vi "Mark as Source Only.vi"() -> ()   [LabVIEW 2011]
uses:
  <vilib>/regexp/Match Regular Expression.xnode
panel:
  out "Array":path[](array[path])
  out "Progess":i32(slide) scale=0.0..20.0
  in  "Mark VIs":bool
  in  "IgnoreSVN":bool=TRUE
  in  "Root Folder":path
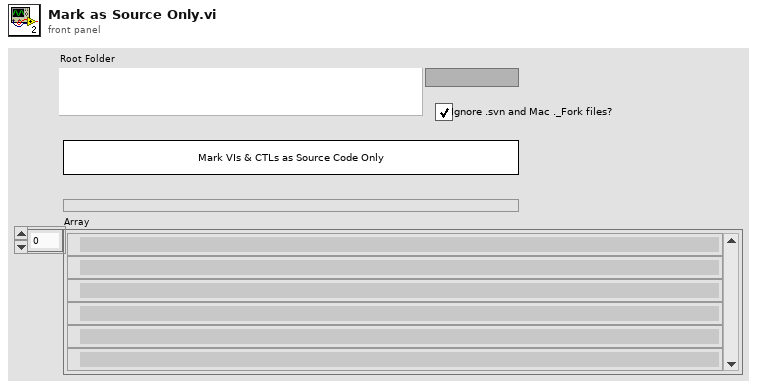
[diagram p1: front panel]
types:
  T1 = enum32{"invalid VI type", "Standard VI", "Control VI", "Global VI", "Polymorphic VI", "Configuration VI", "SubSystem", "Facade VI", "Method VI", "Statechart Diagram VI"}[]
  T2 = enum32{"invalid VI type", "Standard VI", "Control VI", "Global VI", "Polymorphic VI", "Configuration VI", "SubSystem", "Facade VI", "Method VI", "Statechart Diagram VI"}
  T3 = enum16{"Left Button", "Center Button", "Right Button", "Window Close"}
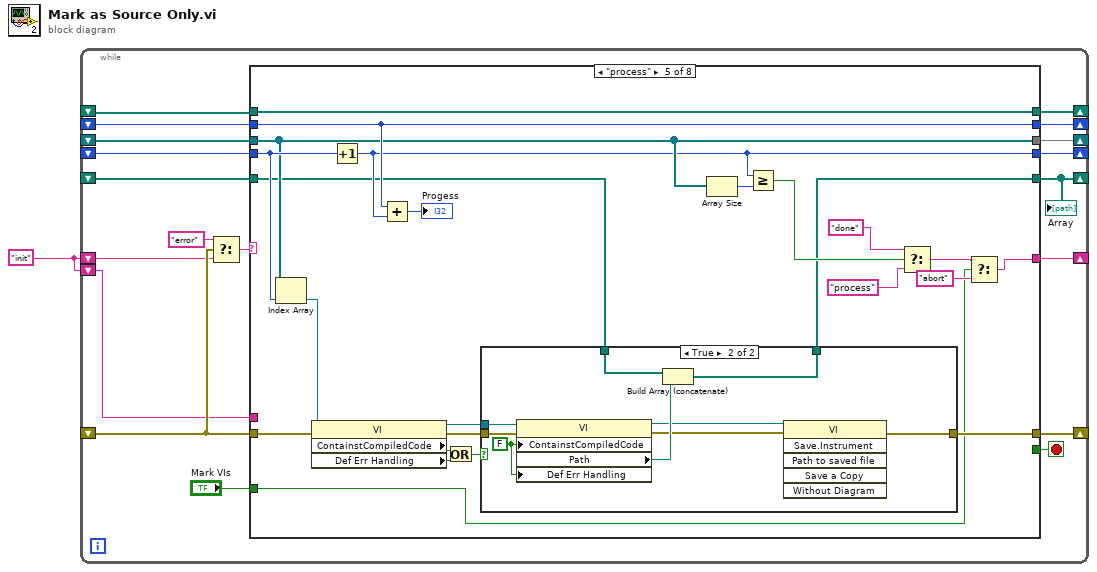
[diagram p0: block diagram]
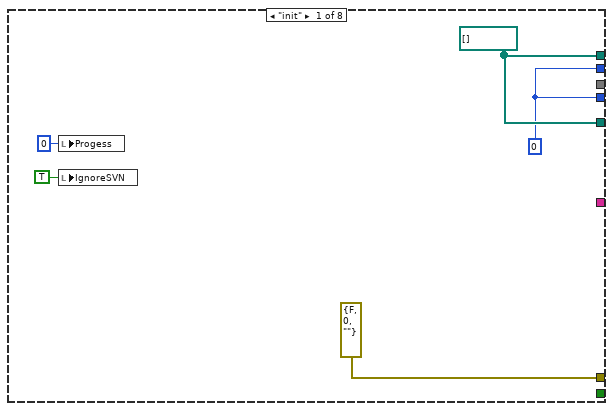
[diagram p2: hidden frame]
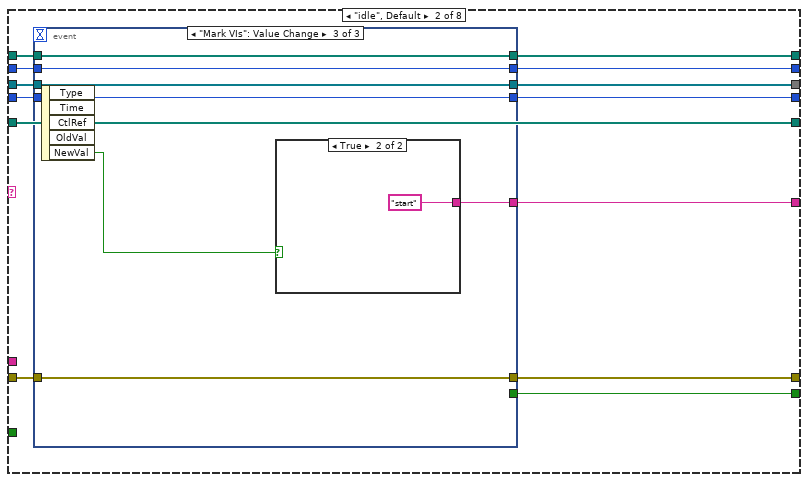
[diagram p3: hidden frame]
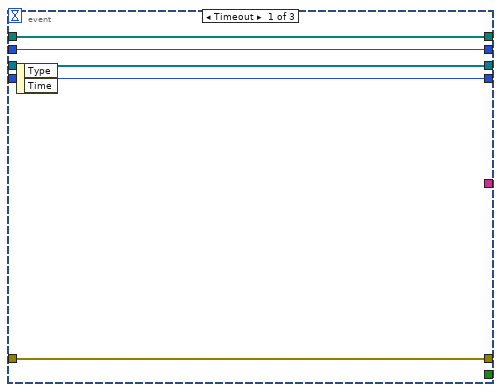
[diagram p4: hidden frame]
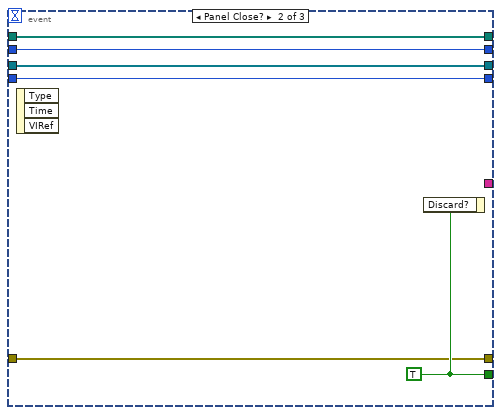
[diagram p5: hidden frame]
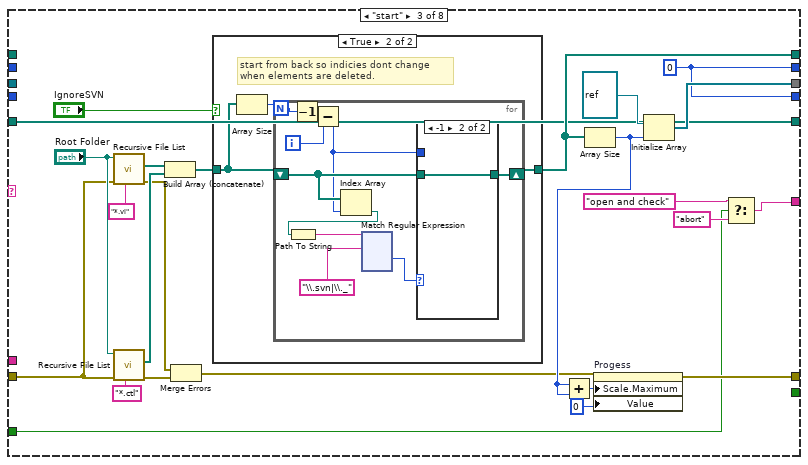
[diagram p7: hidden frame]
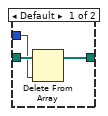
[diagram p9: hidden frame]
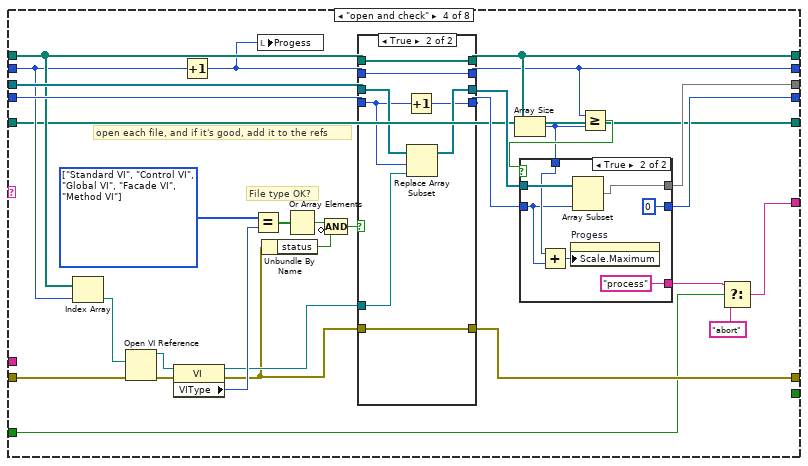
[diagram p10: hidden frame]
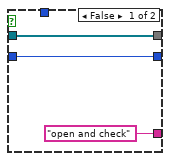
[diagram p11: hidden frame]
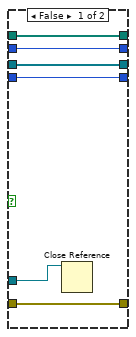
[diagram p12: hidden frame]
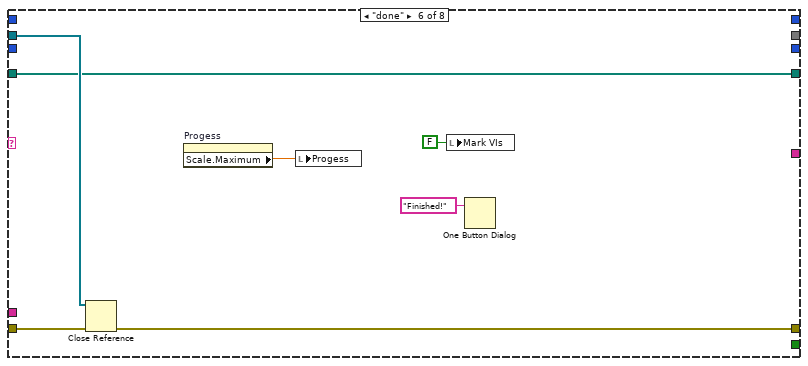
[diagram p14: hidden frame]
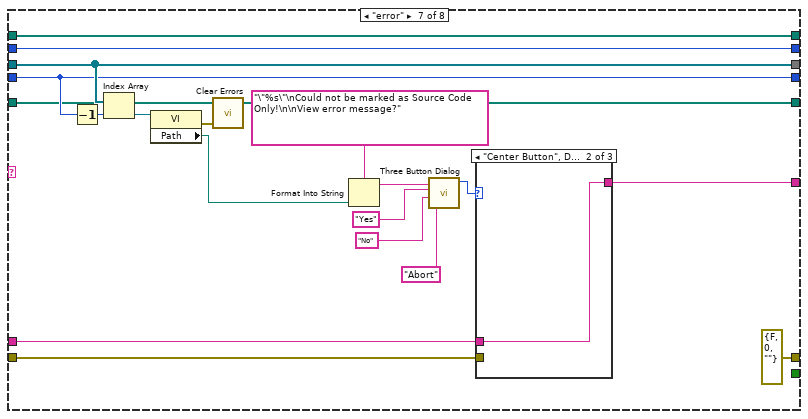
[diagram p15: hidden frame]
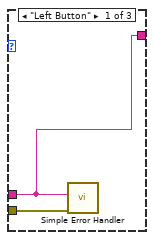
[diagram p16: hidden frame]
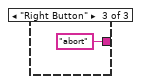
[diagram p17: hidden frame]
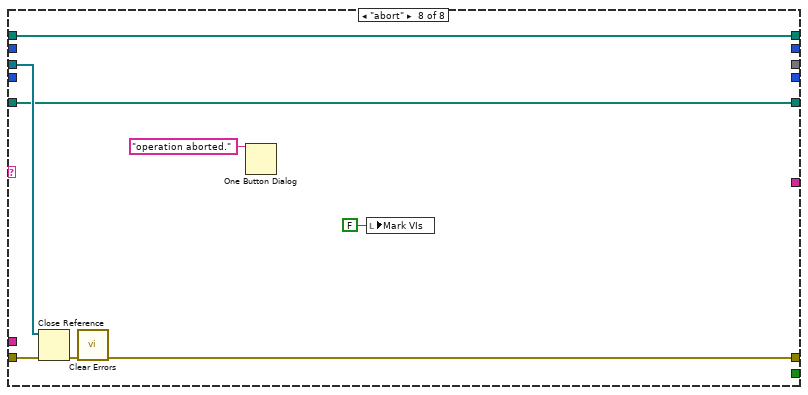
[diagram p18: hidden frame]
diagram:
  w1 = "init"
  n1 = while {
    shift-right: [w15] -> _
    shift-left: w1 -> [w4]
    shift-right: [w16] -> _
    shift-left: _ -> [w17]
    shift-right: [w14] -> _
    shift-left: _ -> [w13]
    shift-right: [w11] -> _
    shift-left: _ -> [w12]
    shift-right: [w10] -> _
    shift-left: _ -> [w9]
    shift-right: [w7] -> _
    shift-left: _ -> [w8]
    shift-left: w1 -> [w5]
    shift-right: [w2] -> _
    shift-left: _ -> [w3]
    stop <- w20 stop-if-true
    n2 = Select(t="error", s=w17, f=w4) -> (s? t:f=w18:string)
    n3 = case shown="\"process\"" w18 {
      tunnel: [_ w38 _ _ _ _ _ _] -> w20
      tunnel: w17 -> [_ w37 w67 w241 w273 w307 w317 w335]
      tunnel: [errorcluster {"status"=FALSE, "code"=0, "source"=""} ("error in") w36 w76 w227 w285 w305 errorcluster {"status"=FALSE, "code"=0, "source"=""} ("error out") w333] -> w16
      tunnel: [_ w35 w60 w213 w277 _ w312 _] -> w15
      tunnel: [w23 w32 w63 w224 w286 _ w326 w332] -> w14
      tunnel: w13 -> [_ w34 _ w228 w286 _ w326 w332]
      tunnel: w12 -> [_ w33 _ w225 w287 _ w325 _]
      tunnel: [w22 w31 w70 w220 w287 _ w325 _] -> w11
      tunnel: [_ w30 w73 w218 w284 _ w323 _] -> w10
      tunnel: w9 -> [_ w29 _ w234 w284 w306 w323 w336]
      tunnel: w8 -> [_ w28 _ w232 w289 _ w311 _]
      tunnel: [w22 w27 w70 w221 w282 _ w311 _] -> w7
      tunnel: "Mark VIs" -> [_ _ w59 w215 w275 _ _ _]
      tunnel: w5 -> [_ _ _ _ _ _ w309 _]
      tunnel: w3 -> [_ w26 w58 w211 w270 w301 w308 w331]
      tunnel: [w23 w26 w58 w211 w269 w301 w308 w331] -> w2
      frame "init" {
        w22 = 0
        w23 = path[] []
        n4 = local write "Progess"(0 ("Progess")) -> ()
        n5 = local write "IgnoreSVN"(TRUE ("IgnoreSVN")) -> ()
      }
      frame "idle", Default {
        n6 = event shown="[2] \"Mark VIs\": Value Change" {
          selector: _ -> [_ _ _]
          dyn-events: _ -> [_ _ _]
          timeout: _ -> [_ _ _]
          tunnel: [_ w49 _] -> w38
          tunnel: w37 -> [w43 w48 w56]
          tunnel: [w43 w48 w56] -> w36
          tunnel: [_ _ w55] -> w35
          tunnel: w34 -> [w41 w47 w53]
          tunnel: w33 -> [w42 w46 w54]
          tunnel: [w41 w47 w53] -> w32
          tunnel: [w42 w46 w54] -> w31
          tunnel: [w39 w45 w51] -> w30
          tunnel: w29 -> [w39 w45 w51]
          tunnel: w28 -> [w40 w44 w52]
          tunnel: [w40 w44 w52] -> w27
          event Timeout {
            n7 = event-data() -> ()  [unwired: 1 in, 2 out]
          }
          event Panel Close? {
            w49 = TRUE
            n8 = event-data() -> ()  [unwired: 1 in, 3 out]
            n9 = event-data("Discard?"=w49) -> ()  [unwired: 1 in, 1 out]
          }
          event "Mark VIs": Value Change {
            n10 = event-data() -> ("NewVal"=w50:bool)  [unwired: 1 in, 4 out]
            n11 = case shown="True" w50 {
              tunnel: [_ "start"] -> w55
              frame False {
              }
              frame True {
              }
            }
          }
        }
      }
      frame "start" {
        w70 = 0
        n12 = call <vilib>:"Recursive File List.vi"("pattern"="*.vi", "error in (no error)"=w67, "Folder Path"="Root Folder") -> ("error out"=w68:errorcluster, "All Files in Dir"=w78:path[])  [unwired: 4 in, 3 out]
        n13 = call <vilib>:"Recursive File List.vi"("pattern"="*.ctl", "error in (no error)"=w67, "Folder Path"="Root Folder") -> ("error out"=w66:errorcluster, "All Files in Dir"=w77:path[])  [unwired: 4 in, 3 out]
        n14 = Build Array (concatenate)(w78, w77) -> (w69:path[])
        n15 = Merge Errors(w68, w66) -> (w65:errorcluster)
        n16 = case shown="True" "IgnoreSVN" {
          tunnel: w69 -> [w82 w83]
          tunnel: [w82 w85] -> w63
          frame False {
          }
          frame True {
            # "start from back so indicies dont change\nwhen elements are deleted."
            n17 = Array Size(array=w83) -> (size(s)=w84:i32)
            n18 = for {
              N: w84 -> [w95]
              shift-right: [w90] -> w85
              shift-left: w83 -> [w92]
              i -> [w94]
              n19 = Decrement(x=w95) -> (x-1=w89:i32)
              n20 = Subtract(x=w89, y=w94) -> (x-y=w91:i32)
              n21 = Index Array(array=w92, index=w91) -> (element=w93:path)
              n22 = Path To String(path=w93) -> (string=w88:string)
              n23 = xnode "Match Regular Expression"("input string"=w88, "regular expression"="\\.svn|\\._") -> ("offset past match"=w87:i32)  [unwired: 4 in, 4 out]
              n24 = case shown="-1" w87 {
                tunnel: w92 -> [w209 w210]
                tunnel: w91 -> [w207 _]
                tunnel: [w208 w210] -> w90
                frame Default {
                  n25 = Delete From Array(array=w209, index=w207) -> (array with subset deleted=w208:path[])  [unwired: 1 in, 1 out]
                }
                frame -1 {
                }
              }
            }
          }
        }
        n26 = Array Size(array=w63) -> (size(s)=w71:i32)
        n27 = Add(x=w71, y=w71) -> (x+y=w72:i32)
        n28 = property on="Progess" class="Slide (strict)"(error in=w65, "Scale.Maximum"=w72, "Value"=0 ("Progess")) -> (error out=w76:errorcluster)  [unwired: 1 in, 1 out]
        n29 = Initialize Array(refnum<vi> refnum ("This VI"), w71) -> (w73:refnum<vi>[])
        n30 = Select(t="open and check", s=w59, f="abort") -> (s? t:f=w60:string)
      }
      frame "open and check" {
        w236 = T1 [enum."Standard VI", enum."Control VI", enum."Global VI", enum."Facade VI", enum."Method VI"] items=["invalid VI type", "Standard VI", "Control VI", "Global VI", "Polymorphic VI", "Configuration VI", "SubSystem", "Facade VI", "Method VI", "Statechart Diagram VI"]
        # "open each file, and if it's good, add it to the refs"
        # "File type OK?"
        n31 = Index Array(array=w228, index=w225) -> (element=w240:path)
        n32 = Open VI Reference(vi path=w240, error in (no error)=w241) -> (vi reference=w238:refnum<vi>, error out=w239:errorcluster)  [unwired: 4 in]
        n33 = property class="VI"(reference=w238, error in=w239) -> (reference out=w233:refnum<vi>, error out=w226:errorcluster, "VIType"=w237:T2)
        n34 = Increment(x=w225) -> (x+1=w219:i32)
        n35 = Equal?(x=w236, y=w237) -> (x = y?=w235:bool[])
        n36 = local write "Progess"(w219) -> ()
        n37 = Unbundle By Name(w226) -> ("status"=w230:bool)
        n38 = Or Array Elements(Boolean array=w235) -> (logical OR=w231:bool)
        n39 = Compound Arithmetic op=AND(w231, invert w230) -> (w229:bool)
        n40 = case shown="True" w229 {
          tunnel: w234 -> [w255 w265]
          tunnel: w233 -> [w253 w264]
          tunnel: [w255 w263] -> w222
          tunnel: w232 -> [w254 w262]
          tunnel: [w254 w261] -> w217
          tunnel: w228 -> [w257 w260]
          tunnel: [w257 w260] -> w224
          tunnel: [w256 w259] -> w220
          tunnel: w219 -> [w256 w259]
          tunnel: [w252 w258] -> w227
          tunnel: w226 -> [w252 w258]
          frame False {
            n41 = Close Reference(reference=w253) -> ()  [unwired: 1 in, 1 out]
          }
          frame True {
            n42 = Increment(x=w262) -> (x+1=w261:i32)
            n43 = Replace Array Subset(array=w265, new element=w264, index=w262) -> (w263:refnum<vi>[])
          }
        }
        n44 = Array Size(array=w224) -> (size(s)=w216:i32)
        n45 = Greater Or Equal?(x=w220, y=w216) -> (x >= y?=w223:bool)
        n46 = case shown="True" w223 {
          tunnel: w222 -> [w244 w249]
          tunnel: w217 -> [w243 w245]
          tunnel: [w244 w248] -> w218
          tunnel: [w243 0] -> w221
          tunnel: ["open and check" "process"] -> w212
          tunnel: w216 -> [_ w246]
          frame False {
          }
          frame True {
            n47 = Add(x=w246, y=w245) -> (x+y=w250:i32)
            n48 = property on="Progess" class="Slide (strict)"("Scale.Maximum"=w250) -> ()  [unwired: 2 in, 2 out]
            n49 = Array Subset(array=w249, length=w245) -> (w248:refnum<vi>[])  [unwired: 1 in]
          }
        }
        n50 = Select(t=w212, s=w215, f="abort") -> (s? t:f=w213:string)
      }
      frame "process" {
        n51 = Index Array(array=w284, index=w289) -> (element=w274:refnum<vi>)
        n52 = property class="VI"(reference=w274, error in=w273) -> (reference out=w272:refnum<vi>, error out=w271:errorcluster, "ContainstCompiledCode"=w267:bool, "Def Err Handling"=w266:bool)
        n53 = Increment(x=w289) -> (x+1=w282:i32)
        n54 = Add(x=w287, y=w282) -> (x+y=→"Progess":i32)
        n55 = Or(x=w267, y=w266) -> (x .or. y?=w268:bool)
        n56 = case shown="True" w268 {
          tunnel: [w291 w300] -> w285
          tunnel: w272 -> [_ w299]
          tunnel: w271 -> [w291 w298]
          tunnel: w270 -> [w290 w297]
          tunnel: [w290 w295] -> w269
          frame False {
          }
          frame True {
            w292 = FALSE ("Contains Compiled Code")
            n57 = property class="VI"(reference=w299, error in=w298, "ContainstCompiledCode"=w292, "Def Err Handling"=w292) -> (reference out=w294:refnum<vi>, error out=w293:errorcluster, "Path"=w296:path)
            n58 = Build Array (concatenate)(w297, w296) -> (w295:path[])
            n59 = invoke class="VI" method="Save.Instrument"(reference=w294, error in=w293) -> (error out=w300:errorcluster)  [unwired: 4 in, 5 out]
          }
        }
        n60 = Array Size(array=w284) -> (size(s)=w283:i32)
        n61 = Greater Or Equal?(x=w282, y=w283) -> (x >= y?=w281:bool)
        n62 = Select(t="done", s=w281, f="process") -> (s? t:f=w278:string)
        n63 = Select(t=w278, s=w275, f="abort") -> (s? t:f=w277:string)
      }
      frame "done" {
        n64 = Close Reference(reference=w306, error in (no error)=w307) -> (error out=w305:errorcluster)
        n65 = property on="Progess" class="Slide (strict)"() -> ("Scale.Maximum"=w304:dbl)  [unwired: 2 in, 2 out]
        n66 = local write "Progess"(w304) -> ()
        n67 = local write "Mark VIs"(FALSE ("Mark VIs")) -> ()
        n68 = One Button Dialog(message="Finished!") -> ()  [unwired: 1 in, 1 out]
      }
      frame "error" {
        n69 = Decrement(x=w311) -> (x-1=w322:i32)
        n70 = Index Array(array=w323, index=w322) -> (element=w324:refnum<vi>)
        n71 = property class="VI"(reference=w324) -> (error out=w316:errorcluster, "Path"=w321:path)  [unwired: 1 in, 1 out]
        n72 = call <vilib>:"Clear Errors.vi"("error in (no error)"=w316) -> ()  [unwired: 6 in, 1 out]
        n73 = Format Into String(format string="\"%s\"\nCould not be marked as Source Code Only!\n\nView error message?", w321) -> (resulting string=w319:string)  [unwired: 2 in, 1 out]
        n74 = call <vilib>:"Three Button Dialog.vi"("Right Button Text (\"Cancel\")"="Abort" ("Right Button Text (\"Cancel\")"), "Center Button Text (\"No\")"="No" ("F button name (\"Cancel\")"), "Left Button Text (\"Yes\")"="Yes" ("T button name (\"OK\")"), "message"=w319) -> ("Which Button?"=w318:T3)  [unwired: 7 in]
        n75 = case shown="\"Center Button\", Default" w318 {
          tunnel: w317 -> [w328 _ _]
          tunnel: [w327 w329 "abort"] -> w312
          tunnel: w309 -> [w327 w329 _]
          frame "Left Button" {
            n76 = call <vilib>:"Simple Error Handler.vi"("error source (\" \")"=w327, "error in (no error)"=w328) -> ()  [unwired: 3 in, 5 out]
          }
          frame "Center Button", Default {
          }
          frame "Right Button" {
          }
        }
      }
      frame "abort" {
        n77 = Close Reference(reference=w336, error in (no error)=w335) -> (error out=w334:errorcluster)
        n78 = call <vilib>:"Clear Errors.vi"("error in (no error)"=w334) -> ("error out"=w333:errorcluster)  [unwired: 6 in]
        n79 = One Button Dialog(message="operation aborted.") -> ()  [unwired: 1 in, 1 out]
        n80 = local write "Mark VIs"(FALSE ("Mark VIs")) -> ()
      }
    }
    "Array" <- w2
  }
